vi "Compile Aliases.vi"(8 "error in (no error)":errorcluster, 11 "Device Ref in":T1 format="%.0x") -> (0 "error out":errorcluster, 2 "Alias Mappings":T2[](array[typedef]), 3 "Device Ref out":T1 format="%.0x")   [LabVIEW 2017, in "Routing and Faulting System Explorer.lvlib"]
uses:
  Routing and Faulting System Explorer.lvlib
  Shared/Alias Mapping.ctl
  <vilib>/NI Veristand/Custom Device API/Custom Device Item Ref.ctl
  Shared/Constants.vi
  <vilib>/NI Veristand/Custom Device Tools/Custom Device Utility Library/NI VeriStand - Search for Item by Name.vi
  <vilib>/NI Veristand/Custom Device Tools/Custom Device Utility Library/Custom Device Utility Library.lvlib
  Shared/Routing and Faulting Shared.lvlib
  Scripting/Routing and Faulting Scripting.lvlib
  <vilib>/NI VeriStand/Custom Device API/Custom Device API.lvlib
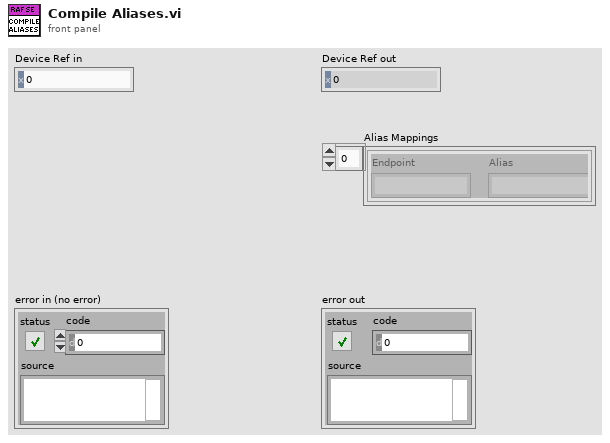
[diagram p1: front panel]
types:
  T1 = typedef "Custom Device API.lvlib/Custom Device Item Ref.ctl" = u64
  T2 = typedef "Routing and Faulting Shared.lvlib/Alias Mapping.ctl" = cluster{"Endpoint":string, "Alias":string}
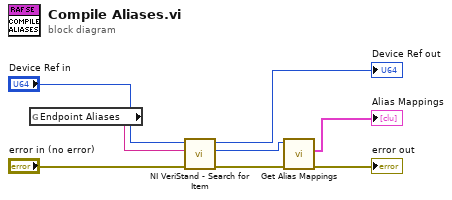
[diagram p0: block diagram]
diagram:
  n1 = global read "Constants.vi" "Endpoint Aliases"() -> (w8:string)
  n2 = call-poly <vilib>:"NI VeriStand - Search for Item.vi"("error in"="error in (no error)", "Item Name"=w8, "Section Ref in"="Device Ref in") -> ("error out"=w3:errorcluster, "Item Ref"=w4:T1, "Section Ref out"=→"Device Ref out":T1)  [unwired: 5 in, 1 out]
  n3 = call "Get Alias Mappings.vi"("error in (no error)"=w3, "Endpoint Aliases Ref in"=w4) -> ("error out"=→"error out":errorcluster, "Alias Mappings"=→"Alias Mappings":T2[])  [unwired: 7 in, 1 out]
